vi "Vector3D Norm.vi"(1 "Vector3D":T1={"Thumb"=[0.0, 0.0, 0.0], "Middle"=[0.0, 0.0, 0.0], "Index"=[0.0, 0.0, 0.0]}) -> (0 "Vectors Norm":dbl[](array[numeric]))   [LabVIEW 2013]
uses:
  controls/Vector3D Fingers.ctl
  <vilib>/Analysis/_algsub.llb/Real Vector Norm.vi
  <vilib>/Analysis/NI_AALPro.lvlib
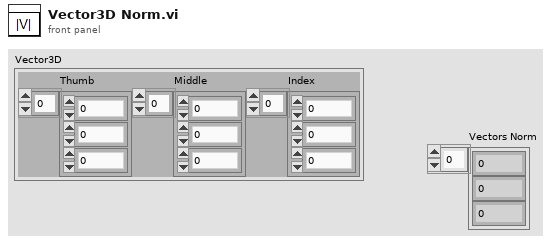
[diagram p1: front panel]
types:
  T1 = typedef "Vector3D Fingers.ctl" = cluster{"Thumb":dbl[], "Middle":dbl[], "Index":dbl[]}
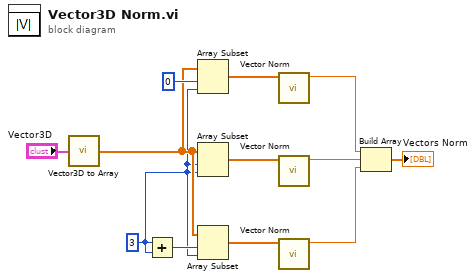
[diagram p0: block diagram]
diagram:
  w3 = 3 ("length")
  n1 = call "Vector3D to Array.vi"("Vector3D"="Vector3D") -> ("Array"=w9:dbl[])
  n2 = Add(x=w3, y=w3) -> (x+y=w4:i32)
  n3 = Array Subset(array=w9, index=0, length=w3) -> (w12:dbl[])
  n4 = Array Subset(array=w9, index=w3, length=w3) -> (w10:dbl[])
  n5 = Array Subset(array=w9, index=w4, length=w3) -> (w8:dbl[])
  n6 = call-poly <vilib>:"Vector Norm.vi"("Input Vector"=w12) -> ("norm"=w7:dbl)  [unwired: 9 in, 1 out]
  n7 = call-poly <vilib>:"Vector Norm.vi"("Input Vector"=w10) -> ("norm"=w6:dbl)  [unwired: 9 in, 1 out]
  n8 = call-poly <vilib>:"Vector Norm.vi"("Input Vector"=w8) -> ("norm"=w5:dbl)  [unwired: 9 in, 1 out]
  n9 = Build Array(w7, w6, w5) -> (→"Vectors Norm":dbl[])
